vi "Fluke 5080 Error Measurement Calibrator.vi"() -> ()   [LabVIEW 2012]
doc: "This example shows how to configure the calibrator to error measurement mode."
uses:
  <instrlib>/Fluke 5080/Fluke 5080.lvlib
panel:
  out "Updated Reference Unit":i32(ring) items=["V", "dBm", "A", "Ohm", "Hz"]
  out "Updated Reference Value":dbl
  out "Original Reference Unit":i32(ring) items=["V", "dBm", "A", "Ohm", "Hz"]
  out "Original Reference Value":dbl
  out "Error Data Unit (0: Threshold 1000)":i32(ring) items=["Result Error"=-1, "Threshold 1000"=0, "Threshold 100"=1, "Threshold 10"=2, "Parts-per-million"=3, "Percent"=4]
  out "Error":dbl
  in  "Adjustment Direction (0: Increment)":i32(ring)=1 items=["Increment", "Decrement"]
  in  "Adjustment Value (0)":dbl=0.25
  in  "Adjustment Type (0: Multiply)":i32(ring)=1 items=["Multiply", "Increments or Decrements"]
  in  "Error Unit (0: Threshold 1000)":i32(ring)=4 items=["Threshold 1000", "Threshold 100", "Threshold 10", "Parts-per-million", "Percent"]
  in  "Serial Configuration":T1={"Baud Rate"=9600, "Parity"=0, "Data Bits"=8, "Stop Bits"=10, "Flow Control"=0} {"Flow Control" items=["None", "XON/XOFF", "RTS/CTS", "XON/XOFF & RTS/CTS", "DTR/DSR", "XON/XOFF & DTR/DSR"]; "Stop Bits" items=["1.0"=10, "1.5"=15, "2.0"=20]; "Data Bits" items=["7"=7, "8"=8]; "Parity" items=["None", "Odd", "Even", "Mark", "Space"]; "Baud Rate" items=["300"=300, "600"=600, "1200"=1200, "2400"=2400, "4800"=4800, "9600"=9600, "19200"=19200]}
  in  "VISA resource name":refnum<visa-resource-name>
  in  "Primary Voltage (5.0)":dbl=3.3
  in  "Output Type (0: DC Volts)":i32(ring) items=["DC Volts", "AC Volts", "DC Current", "AC Current", "DC Power", "AC Power", "Dual DC Volts", "Dual AC Volts", "Resistance"]
  # "(c) 2010 National Instruments.  ALL RIGHTS RESERVED."
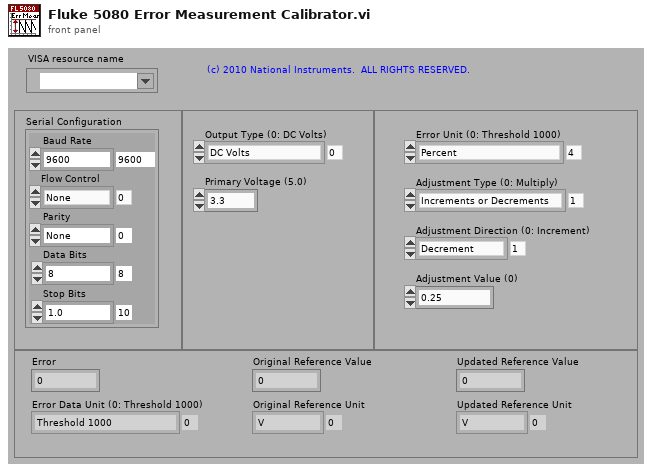
[diagram p1: front panel]
types:
  T1 = cluster{"Baud Rate":u32, "Parity":u16, "Data Bits":u16, "Stop Bits":u16, "Flow Control":u16}
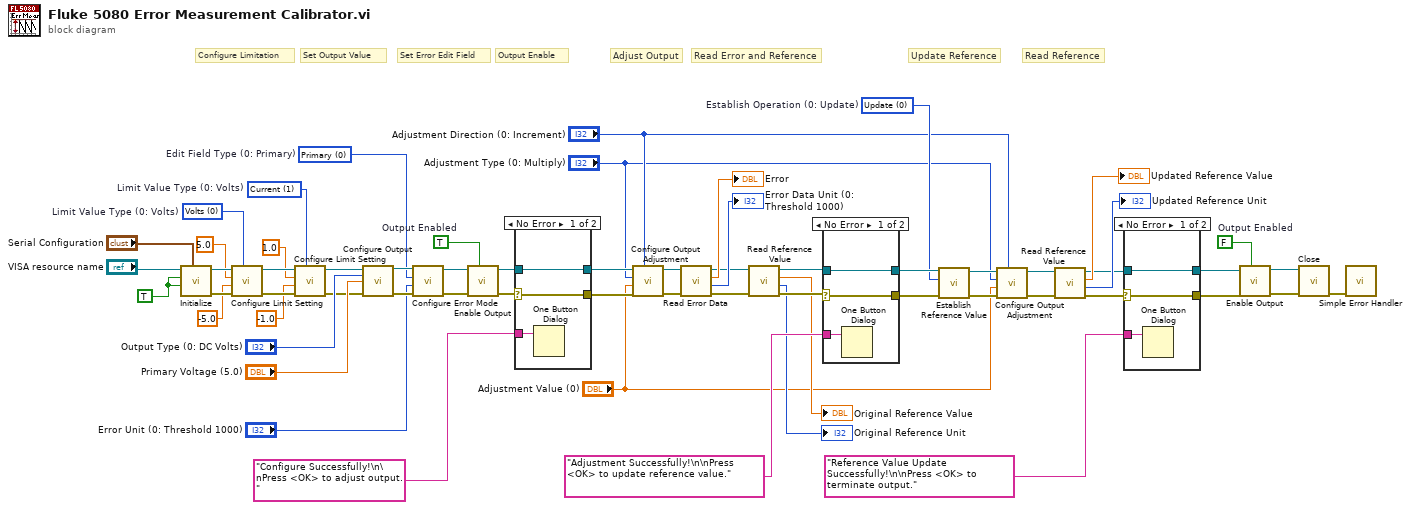
[diagram p0: block diagram]
diagram:
  w3 = 1 items=["Volts", "Current"]  # Limit Value Type (0: Volts)
  w4 = 0 items=["Volts", "Current"]  # Limit Value Type (0: Volts)
  w27 = 0 items=["Update", "Revert"]  # Establish Operation (0: Update)
  w46 = 0 items=["Primary", "Secondary", "Frequency"]  # Edit Field Type (0: Primary)
  w51 = TRUE  # Output Enabled
  w53 = FALSE  # Output Enabled
  w61 = TRUE ("Reset (True)")
  # "Read Reference"
  # "Update Reference"
  # "Read Error and Reference"
  # "Adjust Output"
  # "Output Enable"
  # "Set Error Edit Field"
  # "Set Output Value"
  # "Configure Limitation"
  n1 = call <instrlib>:"Initialize.vi"("Serial Configuration"="Serial Configuration", "Reset (True)"=w61, "ID Query (True)"=w61, "VISA resource name"="VISA resource name") -> ("error out"=w60:errorcluster, "VISA resource name out"=w59:refnum<visa-resource-name>)  [unwired: 1 in, 5 out]
  n2 = call <instrlib>:"Configure Limit Setting.vi"("Limit Value Type (0: Volts)"=w4, "error in (no error)"=w60, "- Limit Value (-5)"=-5.0, "+ Limit Value (5)"=5.0, "VISA resource name"=w59) -> ("error out"=w6:errorcluster, "VISA resource name out"=w8:refnum<visa-resource-name>)  [unwired: 5 out]
  n3 = call <instrlib>:"Configure Limit Setting.vi"("Limit Value Type (0: Volts)"=w3, "error in (no error)"=w6, "- Limit Value (-5)"=-1.0, "+ Limit Value (5)"=1.0, "VISA resource name"=w8) -> ("error out"=w5:errorcluster, "VISA resource name out"=w7:refnum<visa-resource-name>)  [unwired: 5 out]
  n4 = call <instrlib>:"Configure Output.vi"("VISA resource name"=w7, "Output Type (0: DC Volts)"="Output Type (0: DC Volts)", "Primary Voltage (5.0)"="Primary Voltage (5.0)", "error in (no error)"=w5) -> ("VISA resource name out"=w50:refnum<visa-resource-name>, "error out"=w49:errorcluster)  [unwired: 6 in, 4 out]
  n5 = call <instrlib>:"Configure Error Mode.vi"("error in (no error)"=w49, "Error Unit (0: Threshold 1000)"="Error Unit (0: Threshold 1000)", "Edit Field Type (0: Primary)"=w46, "VISA resource name"=w50) -> ("error out"=w47:errorcluster, "VISA resource name out"=w48:refnum<visa-resource-name>)  [unwired: 6 out]
  n6 = call <instrlib>:"Enable Output.vi"("Output Enabled (T: Enable)"=w51, "error in (no error)"=w47, "VISA resource name"=w48) -> ("error out"=w43:errorcluster, "VISA resource name out"=w44:refnum<visa-resource-name>)  [unwired: 7 out]
  n7 = case shown="No Error" w43 {
    selector: w43 -> [w63 w66]
    tunnel: "Configure Successfully!\n\nPress <OK> to adjust output." ("message") -> [w64 _]
    tunnel: [w63 w66] -> w41
    tunnel: [w62 w65] -> w42
    tunnel: w44 -> [w62 w65]
    frame No Error {
      n8 = One Button Dialog(message=w64) -> ()  [unwired: 2 out]
    }
    frame Error {
    }
  }
  n9 = call <instrlib>:"Configure Output Adjustment.vi"("Adjustment Direction (0: Increment)"="Adjustment Direction (0: Increment)", "error in (no error)"=w41, "Adjustment Value (0)"="Adjustment Value (0)", "Adjustment Type (0: Multiply)"="Adjustment Type (0: Multiply)", "VISA resource name"=w42) -> ("error out"=w39:errorcluster, "VISA resource name out"=w40:refnum<visa-resource-name>)  [unwired: 5 out]
  n10 = call <instrlib>:"Read Error Data.vi"("error in (no error)"=w39, "VISA resource name"=w40) -> ("error out"=w35:errorcluster, "Error Unit (0: Threshold 1000)"=→"Error Data Unit (0: Threshold 1000)":i32, "Error"=→"Error":dbl, "VISA resource name out"=w36:refnum<visa-resource-name>)  [unwired: 6 out]
  n11 = call <instrlib>:"Read Reference Value.vi"("error in (no error)"=w35, "VISA resource name"=w36) -> ("error out"=w33:errorcluster, "Reference Unit"=→"Original Reference Unit":i32, "Reference Value"=→"Original Reference Value":dbl, "VISA resource name out"=w34:refnum<visa-resource-name>)  [unwired: 6 out]
  n12 = case shown="No Error" w33 {
    selector: w33 -> [w68 w71]
    tunnel: "Adjustment Successfully!\n\nPress <OK> to update reference value." ("message") -> [w69 _]
    tunnel: [w68 w71] -> w28
    tunnel: [w67 w70] -> w29
    tunnel: w34 -> [w67 w70]
    frame No Error {
      n13 = One Button Dialog(message=w69) -> ()  [unwired: 2 out]
    }
    frame Error {
    }
  }
  n14 = call <instrlib>:"Establish Reference Value.vi"("error in (no error)"=w28, "Establish Operation (0: Update)"=w27, "VISA resource name"=w29) -> ("error out"=w14:errorcluster, "VISA resource name out"=w15:refnum<visa-resource-name>)  [unwired: 7 out]
  n15 = call <instrlib>:"Configure Output Adjustment.vi"("Adjustment Direction (0: Increment)"="Adjustment Direction (0: Increment)", "error in (no error)"=w14, "Adjustment Value (0)"="Adjustment Value (0)", "Adjustment Type (0: Multiply)"="Adjustment Type (0: Multiply)", "VISA resource name"=w15) -> ("error out"=w12:errorcluster, "VISA resource name out"=w13:refnum<visa-resource-name>)  [unwired: 5 out]
  n16 = call <instrlib>:"Read Reference Value.vi"("error in (no error)"=w12, "VISA resource name"=w13) -> ("error out"=w23:errorcluster, "Reference Unit"=→"Updated Reference Unit":i32, "Reference Value"=→"Updated Reference Value":dbl, "VISA resource name out"=w24:refnum<visa-resource-name>)  [unwired: 6 out]
  n17 = case shown="No Error" w23 {
    selector: w23 -> [w73 w76]
    tunnel: "Reference Value Update Successfully!\n\nPress <OK> to terminate output." ("message") -> [w74 _]
    tunnel: [w73 w76] -> w21
    tunnel: [w72 w75] -> w19
    tunnel: w24 -> [w72 w75]
    frame No Error {
      n18 = One Button Dialog(message=w74) -> ()  [unwired: 2 out]
    }
    frame Error {
    }
  }
  n19 = call <instrlib>:"Enable Output.vi"("Output Enabled (T: Enable)"=w53, "error in (no error)"=w21, "VISA resource name"=w19) -> ("error out"=w20:errorcluster, "VISA resource name out"=w18:refnum<visa-resource-name>)  [unwired: 7 out]
  n20 = call <instrlib>:"Close.vi"("error in (no error)"=w20, "VISA resource name"=w18) -> ("error out"=w57:errorcluster)  [unwired: 9 out]
  n21 = call <vilib>:"Simple Error Handler.vi"("error in (no error)"=w57) -> ()  [unwired: 1 in, 8 out]
